vi "lane find.vi"() -> ()   [LabVIEW 2012]
uses:
  G_SEN.vi
  G_NAV.vi
panel:
  out "Waveform Graph 3":dbl[](graph)
  out "XY Graph":cluster{"Y":dbl[], "Y":dbl[]}[](graph)
  out "Waveform Graph 2":dbl[](graph)
  out "Waveform Graph":dbl[](graph)
  out "lane_pt":dbl[][](array[numeric])
  out "lane":dbl[](array[numeric])
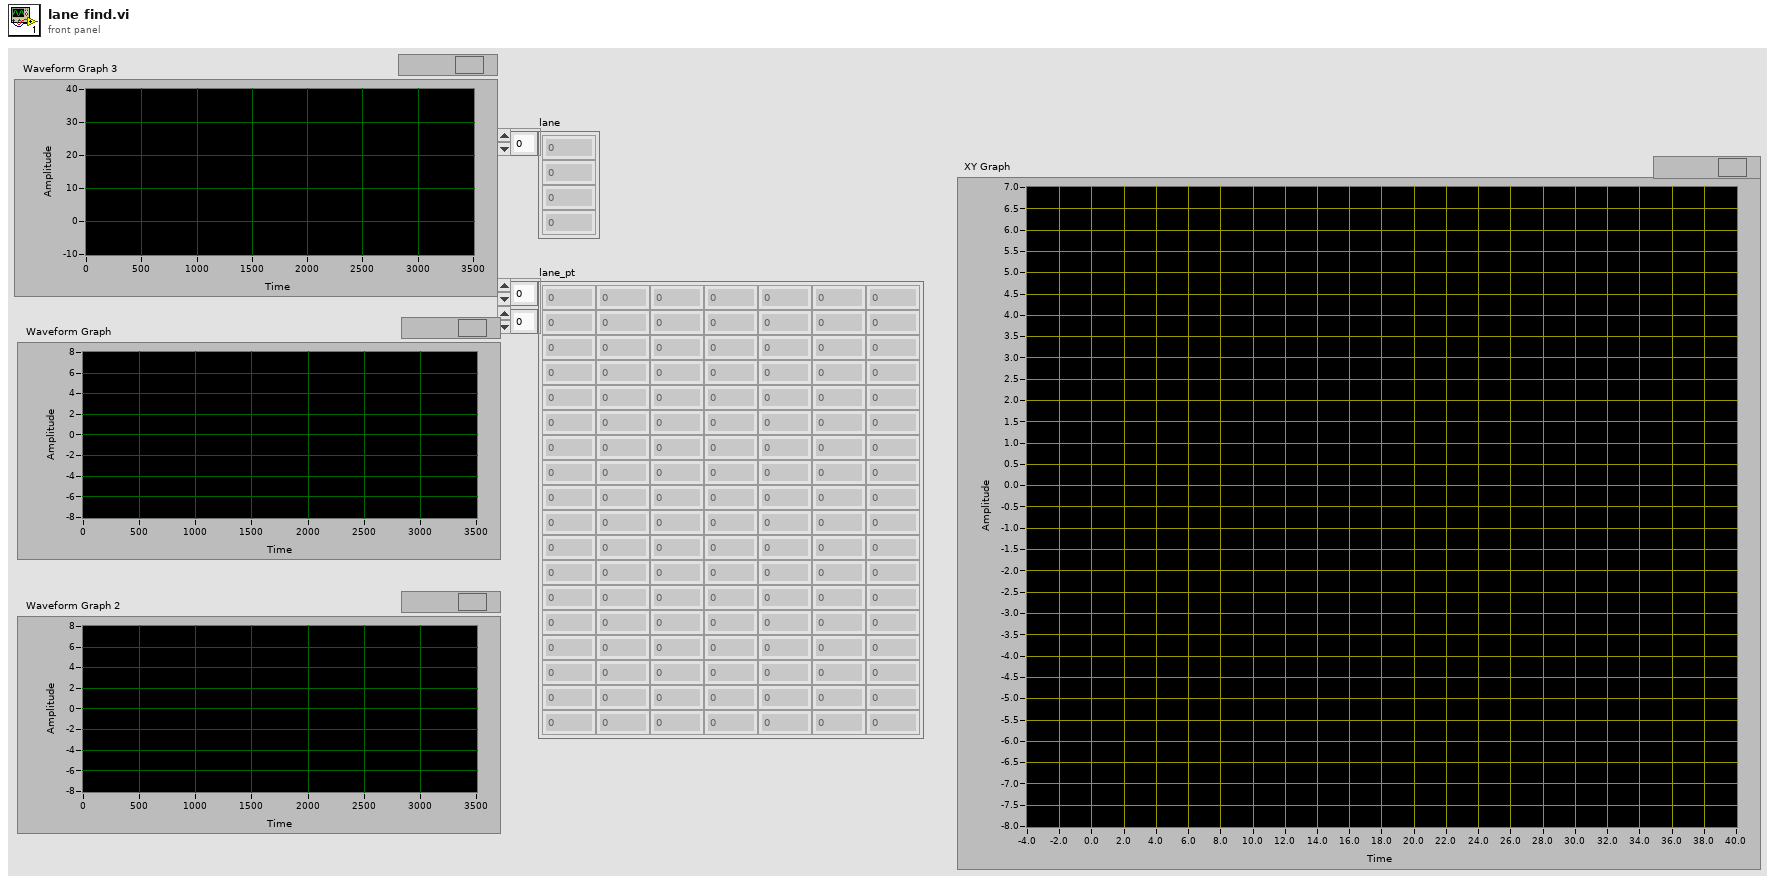
[diagram p1: front panel]
types:
  T1 = cluster{"GPSTime":dbl, "attitude[2]":dbl, "lcc[0]":dbl, "lcc[1]":dbl, "heading_GPS":dbl}
  T2 = cluster{dbl, "element":dbl, "element":dbl, dbl}[]
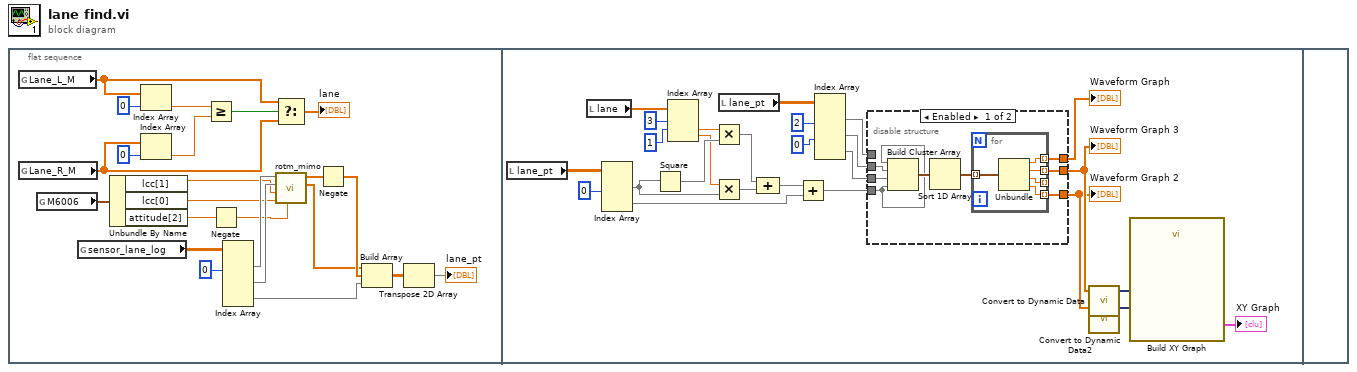
[diagram p0: block diagram]
diagram:
  n1 = flat-sequence {
    frame #0 {
      n2 = global read "G_SEN.vi" "Lane_L_M"() -> (w18:dbl[])
      n3 = global read "G_SEN.vi" "Lane_R_M"() -> (w17:dbl[])
      n4 = global read "G_NAV.vi" "M6006"() -> (w13:T1)
      n5 = global read "G_SEN.vi" "sensor_lane_log"() -> (w8:dbl[][])
      n6 = Unbundle By Name(w13) -> ("lcc[1]"=w9:dbl, "lcc[0]"=w10:dbl, "attitude[2]"=w11:dbl)
      n7 = Index Array(array=w18, index=0) -> (element=w21:dbl)
      n8 = Index Array(array=w17, index=0) -> (element=w20:dbl)
      n9 = Greater Or Equal?(x=w21, y=w20) -> (x >= y?=w19:bool)
      n10 = Negate(x=w11) -> (-x=w12:dbl)
      n11 = Index Array(array=w8, index (col) #1=0 ("disabled index (col)")) -> (element #1=w14:dbl[], element #2=w15:dbl[], element #3=w4:dbl[])  [unwired: 5 in]
      n12 = Select(t=w18, s=w19, f=w17) -> (s? t:f=→"lane":dbl[])
      n13 = call "rotm_mimo.vi"("angle[rad]"=w12, "y0"=w10, "x0"=w9, "y"=w15, "x"=w14) -> ("Y"=w2:dbl[], "X"=w1:dbl[])  [unwired: 3 in, 2 out]
      n14 = Negate(x=w1) -> (-x=w3:dbl[])
      n15 = Build Array(w2, w3, w4) -> (w5:dbl[][])
      n16 = Transpose 2D Array(2D array=w5) -> (transposed array=→"lane_pt":dbl[][])
    }
    frame #1 {
      n17 = local read "lane_pt"() -> (w31:dbl[][])
      n18 = local read "lane"() -> (w48:dbl[])
      n19 = Index Array(array=w31, index (col) #1=0 ("disabled index (col)")) -> (element #1=w30:dbl[], element #2=w27:dbl[])  [unwired: 3 in]
      n20 = Square(x=w30) -> (x^2=w46:dbl[])
      n21 = Index Array(array=w48, index #1=3 ("index"), index #2=1 ("index")) -> (element #2=w45:dbl, element #3=w44:dbl)  [unwired: 1 in, 1 out]
      n22 = Multiply(x=w45, y=w46) -> (x*y=w43:dbl[])
      n23 = Multiply(x=w44, y=w30) -> (x*y=w42:dbl[])
      n24 = local read "lane_pt"() -> (w47:dbl[][])
      n25 = Compound Arithmetic op=ADD(w43, w42) -> (w41:dbl[])
      n26 = Add(x=w41, y=w27) -> (x+y=w25:dbl[])
      n27 = Index Array(array=w47, index (col) #1=2 ("disabled index (col)"), index (col) #2=0 ("index (col)")) -> (element #1=w40:dbl[], element #2=w38:dbl[], element #3=w37:dbl[])  [unwired: 4 in]
      n28 = disable-structure shown="Enabled" {
        disable-tunnel: w40 -> [_ w65]
        disable-tunnel: w38 -> [w57 w64]
        disable-tunnel: w37 -> [w56 _]
        disable-tunnel: [w53 w65] -> w36
        disable-tunnel: [w52 w64] -> w28
        disable-tunnel: w25 -> [w50 w63]
        disable-tunnel: [w51 w63] -> w24
        frame Enabled {
          n29 = Build Cluster Array(w50, w57, w56, w50) -> (w55:T2)
          n30 = Sort 1D Array(array=w55) -> (sorted array=w54:T2)
          n31 = for {
            tunnel: w54 -> [w62] mode=indexing
            tunnel: [w61] -> w53 mode=indexing
            tunnel: [w60] -> w52 mode=indexing
            tunnel: [w59] -> _ mode=indexing
            tunnel: [w58] -> w51 mode=indexing
            n32 = Unbundle(w62) -> (w61:dbl, "element"=w60:dbl, "element"=w59:dbl, w58:dbl)
          }
        }
        frame Disabled {
        }
      }
      "Waveform Graph" <- w36
      "Waveform Graph 2" <- w24
      "Waveform Graph 3" <- w28
      n33 = call "Convert to Dynamic Data"("Array"=w28) -> ("Dynamic Data Type"=w34:dynamicdata)  [unwired: 3 in]
      n34 = call "Convert to Dynamic Data2"("Array"=w24) -> ("Dynamic Data Type"=w33:dynamicdata)  [unwired: 3 in]
      n35 = call "Build XY Graph"("Y Input"=w33, "X Input"=w34) -> ("XY Graph"=→"XY Graph":cluster{"Y":dbl[], "Y":dbl[]}[])  [unwired: 3 in, 6 out]
    }
    frame #2 {
    }
  }
